vi "Lab05.vi"() -> ()   [LabVIEW 2022 SP3]
uses:
  <vilib>/Utility/file.llb/Read Delimited Spreadsheet (DBL).vi
panel:
  out "size(s)":i32
  out "Phase":dbl
  out "Waveform Graph":dbl[](graph)
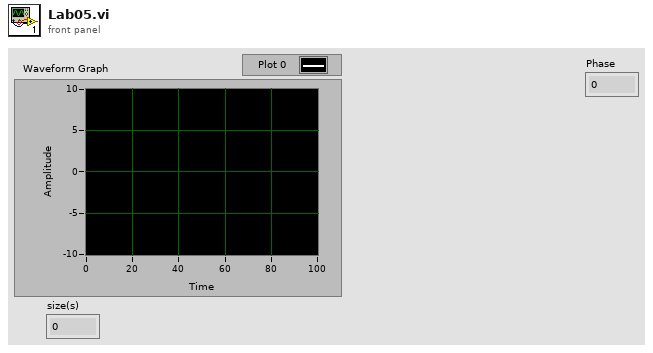
[diagram p1: front panel]
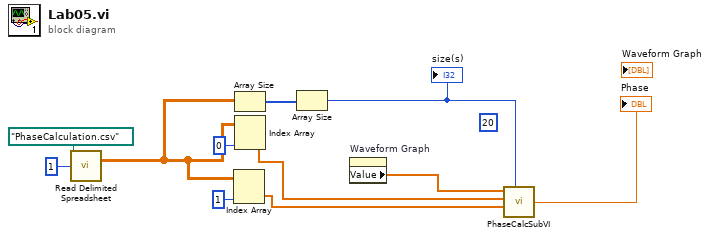
[diagram p0: block diagram]
diagram:
  (unwired) 20 ("Number of Points/Period")
  n1 = call-poly <vilib>:"Read Delimited Spreadsheet.vi"("file path (dialog if empty)"=path "PhaseCalculation.csv", "start of read offset (chars.:0)"=1) -> ("all rows"=w4:dbl[][])  [unwired: 8 in, 5 out]
  n2 = Index Array(array=w4, index (col)=1 ("disabled index (col)")) -> (element=w6:dbl[])  [unwired: 1 in]
  n3 = Array Size(array=w4) -> (size(s)=w3:i32[])
  n4 = Index Array(array=w4, index (col)=0 ("disabled index (col)")) -> (element=w5:dbl[])  [unwired: 1 in]
  n5 = Array Size(array=w3) -> (size(s)=w2:i32)
  "size(s)" <- w2
  n6 = property on="Waveform Graph" class="WFGraph (strict)"() -> ("Value"=w1:dbl[])  [unwired: 2 in, 2 out]
  n7 = call "PhaseCalcSubVI.vi"("Reference In"=w1, "Wave_1"=w5, "Wave_2"=w6, "Number of Points/Period"=w2) -> ("Phase"=→"Phase":dbl)  [unwired: 3 in]
